vi "Get_JSON_data.vi"() -> ()   [LabVIEW 2024]
panel:
  out "label":string
  out "confidence":i32
  out "detection_type":string
  out "crop_path":string
  out "Coordonnées\n Rectangles":dbl[](array[numeric])
  in  "index\n detections":i32
  out "element":T1
  out "detection":T2(array[cluster])
  out "annotated_image":string
  out "cluster json":T3
  in  "path":path
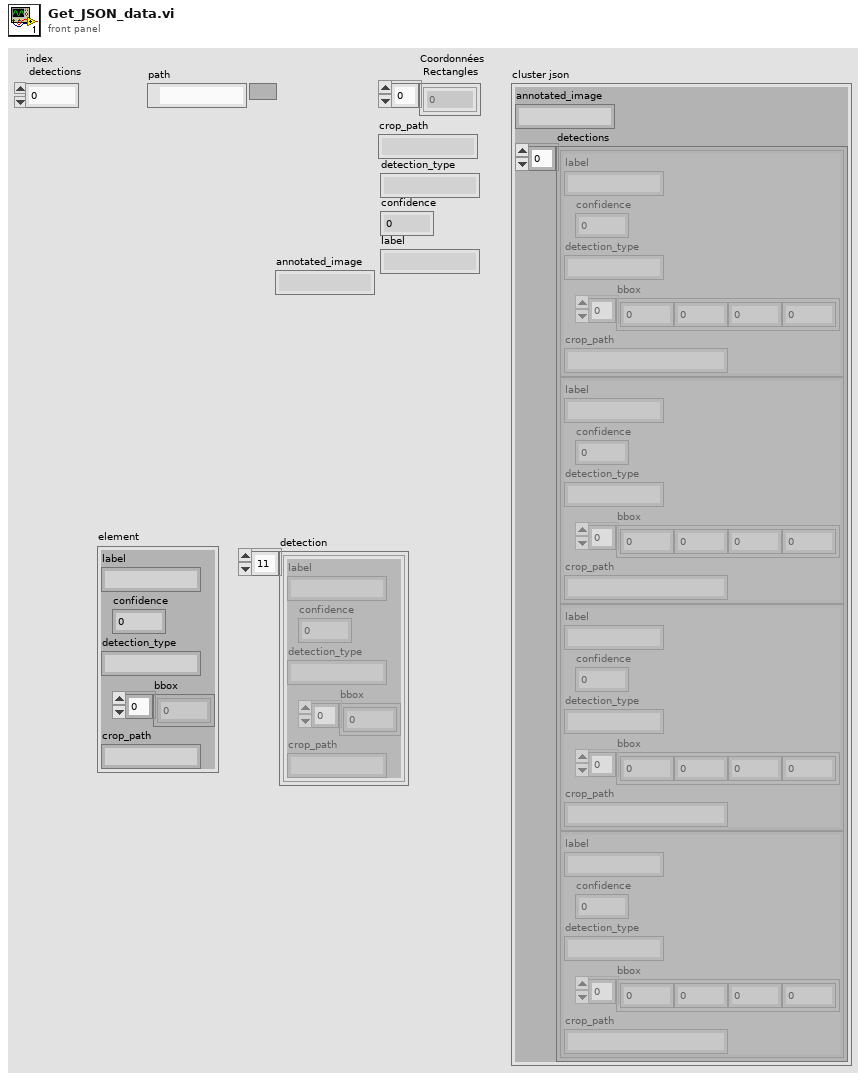
[diagram p1: front panel]
types:
  T1 = cluster{"label":string, "confidence":i32, "detection_type":string, "bbox":dbl[], "crop_path":string}
  T2 = cluster{"label":string, "confidence":i32, "detection_type":string, "bbox":dbl[], "crop_path":string}[]
  T3 = cluster{"annotated_image":string, "detections":cluster{"label":string, "confidence":i32, "detection_type":string, "bbox":dbl[], "crop_path":string}[]}
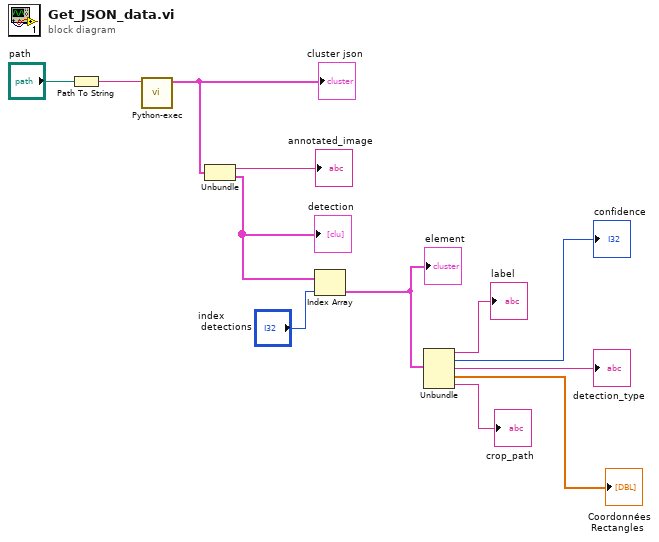
[diagram p0: block diagram]
diagram:
  n1 = Path To String(path="path") -> (string=w11:string)
  n2 = call "Python-exec.vi"("String"=w11) -> ("value"=w10:T3)  [unwired: 10 in]
  "cluster json" <- w10
  n3 = Unbundle(w10) -> ("annotated_image"=→"annotated_image":string, "detections"=w8:T2)
  "detection" <- w8
  n4 = Index Array(array=w8, index="index\n detections") -> (element=w6:T1)
  "element" <- w6
  n5 = Unbundle(w6) -> ("label"=→"label":string, "confidence"=→"confidence":i32, "detection_type"=→"detection_type":string, "bbox"=→"Coordonnées\n Rectangles":dbl[], "crop_path"=→"crop_path":string)
